vi "StoreHeaderMotorInfo.vi"(0 "Temperature":dbl, 1 "StartTime":dbl, 2 "MirrorTrans":dbl, 3 "ROI/Binning String":string, 4 "Anode":i32, 5 "Throwaway Frames":u32, 6 "MirrorAngle":dbl, 7 "error in (no error)":errorcluster, 8 "Image Path":path, 9 "Number of Images":u32, 11 "CameraX":dbl, 12 "ADC speed (kHz)":i32, 13 "Exposure":dbl, 14 "Polarization":dbl, 15 "StartSec":dbl, 16 "EndTime":dbl, 17 "Date String":string, 19 "EndSec":dbl, 20 "Aperture":dbl, 21 "GratingAngle":dbl, 23 "GratingY":dbl, 24 "GratingX":dbl, 25 "Time String":string, 27 "CameraY":dbl) -> ()   [LabVIEW 2015]
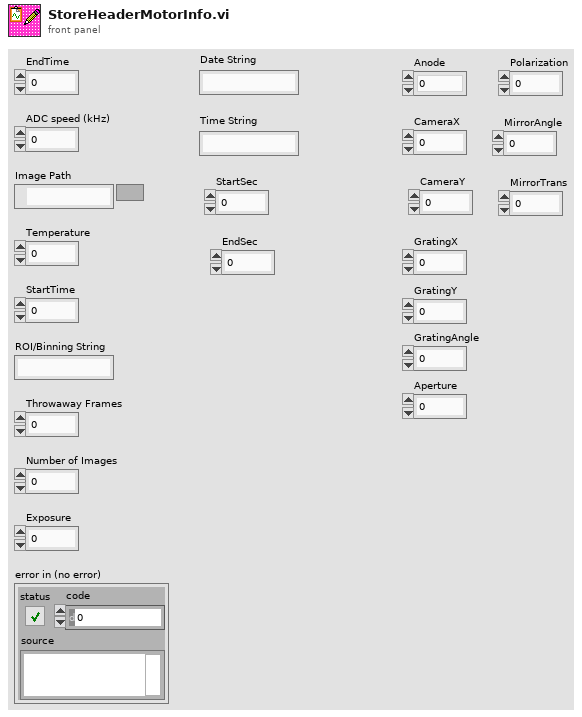
[diagram p1: front panel]
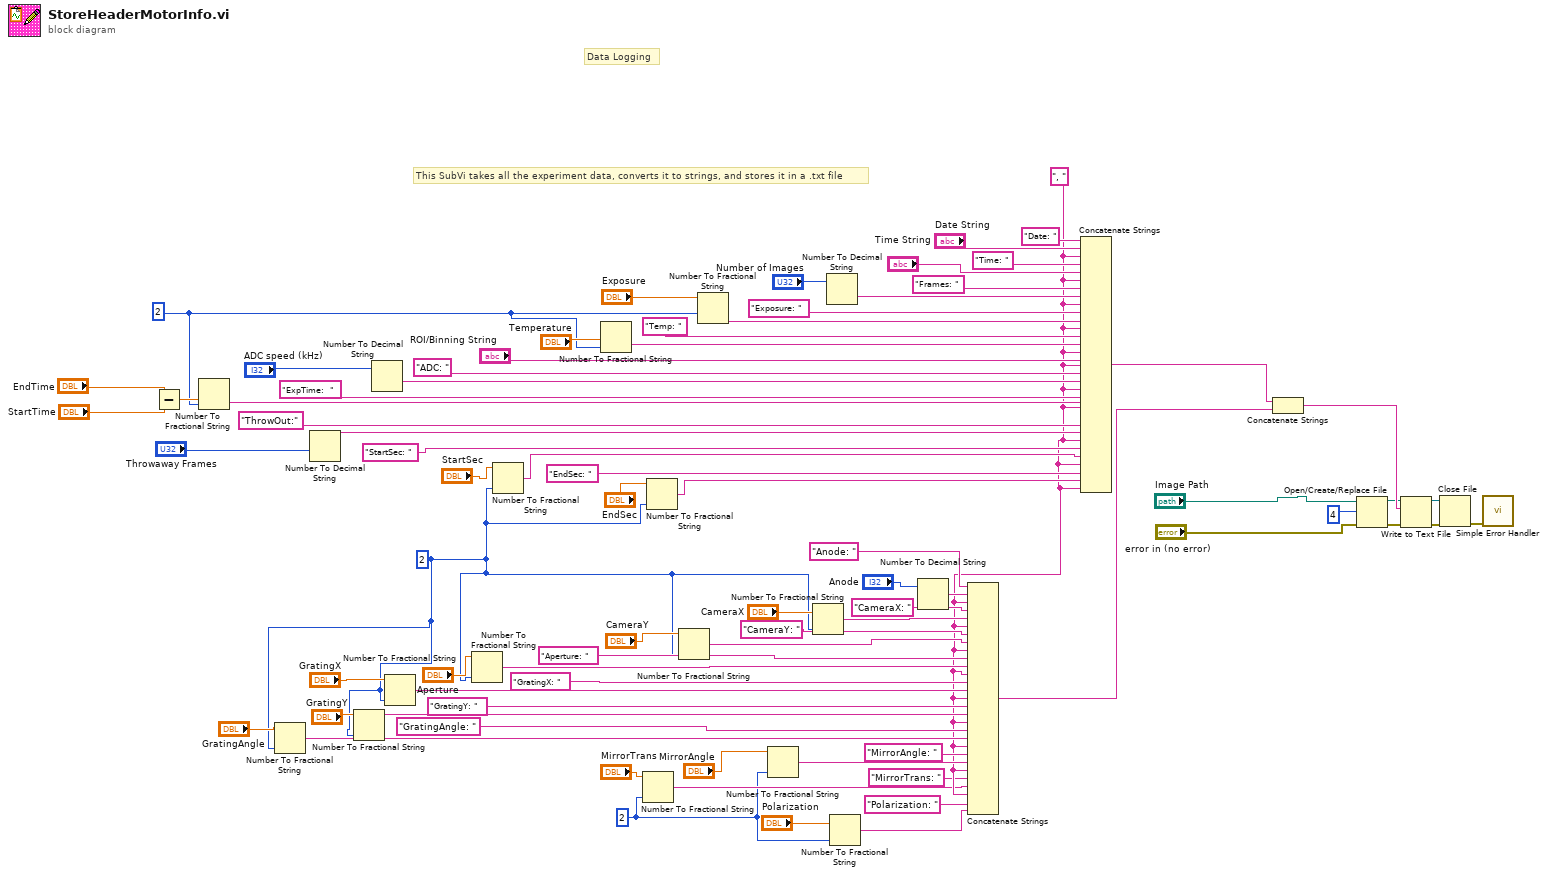
[diagram p0: block diagram]
diagram:
  w3 = 2
  w4 = 2
  w5 = 2
  w17 = ", "
  # "This SubVi takes all the experiment data, converts it to strings, and stores it in a .txt file"
  # "Data Logging"
  n1 = Subtract(x="EndTime", y="StartTime") -> (x-y=w67:dbl)
  n2 = Number To Fractional String(number=w67, precision (6)=w5) -> (F-format string=w70:string)  [unwired: 2 in]
  n3 = Number To Fractional String(number="GratingAngle", precision (6)=w4) -> (F-format string=w21:string)  [unwired: 2 in]
  n4 = Number To Decimal String(number="Throwaway Frames") -> (decimal integer string=w75:string)  [unwired: 1 in]
  n5 = Number To Fractional String(number="GratingY", precision (6)=w4) -> (F-format string=w24:string)  [unwired: 2 in]
  n6 = Number To Decimal String(number="ADC speed (kHz)") -> (decimal integer string=w59:string)  [unwired: 1 in]
  n7 = Number To Fractional String(number="GratingX", precision (6)=w4) -> (F-format string=w27:string)  [unwired: 2 in]
  n8 = Number To Fractional String(number="Aperture", precision (6)=w4) -> (F-format string=w30:string)  [unwired: 2 in]
  n9 = Number To Fractional String(number="StartSec", precision (6)=w4) -> (F-format string=w44:string)  [unwired: 2 in]
  n10 = Number To Fractional String(number="Temperature", precision (6)=w5) -> (F-format string=w55:string)  [unwired: 2 in]
  n11 = Number To Fractional String(number="MirrorTrans", precision (6)=w3) -> (F-format string=w15:string)  [unwired: 2 in]
  n12 = Number To Fractional String(number="EndSec", precision (6)=w4) -> (F-format string=w42:string)  [unwired: 2 in]
  n13 = Number To Fractional String(number="CameraY", precision (6)=w4) -> (F-format string=w33:string)  [unwired: 2 in]
  n14 = Number To Fractional String(number="Exposure", precision (6)=w5) -> (F-format string=w66:string)  [unwired: 2 in]
  n15 = Number To Fractional String(number="MirrorAngle", precision (6)=w3) -> (F-format string=w18:string)  [unwired: 2 in]
  n16 = Number To Fractional String(number="CameraX", precision (6)=w4) -> (F-format string=w36:string)  [unwired: 2 in]
  n17 = Number To Decimal String(number="Number of Images") -> (decimal integer string=w51:string)  [unwired: 1 in]
  n18 = Number To Fractional String(number="Polarization", precision (6)=w3) -> (F-format string=w11:string)  [unwired: 2 in]
  n19 = Number To Decimal String(number="Anode") -> (decimal integer string=w39:string)  [unwired: 1 in]
  n20 = Concatenate Strings("Anode: ", w39, w17, "CameraX: ", w36, w17, "CameraY: ", w33, w17, "Aperture: ", w30, w17, "GratingX: ", w27, w17, "GratingY: ", w24, w17, "GratingAngle: ", w21, w17, "MirrorAngle: ", w18, w17, "MirrorTrans: ", w15, w17, "Polarization: ", w11) -> (w9:string)
  n21 = Concatenate Strings("Date: ", "Date String", w17, "Time: ", "Time String", w17, "Frames: ", w51, w17, "Exposure: ", w66, w17, "Temp: ", w55, w17, "ROI/Binning String", w17, "ADC: ", w59, w17, "ExpTime:  ", w70, w17, "ThrowOut:", w75, w17, "StartSec: ", w44, w17, "EndSec: ", w42, w17) -> (w10:string)
  n22 = Concatenate Strings(w10, w9) -> (w8:string)
  n23 = Open/Create/Replace File(file path (use dialog)="Image Path", error in="error in (no error)", operation (0:open)=4) -> (error out=w62:errorcluster)  [unwired: 3 in, 2 out]
  n24 = Write to Text File(file (use dialog)="Image Path", text=w8, error in=w62) -> (refnum out=w63:refnum<file>, error out=w64:errorcluster)  [unwired: 1 in, 1 out]
  n25 = Close File(refnum=w63, error in=w64) -> (error out=w65:errorcluster)  [unwired: 1 out]
  n26 = call <vilib>:"Simple Error Handler.vi"("error in (no error)"=w65) -> ()  [unwired: 4 in, 5 out]
